vi "Camera Control.vi"(1 "i":i32) -> ()   [LabVIEW 2012]
uses:
  <vilib>/Rock Robotics/WPI/Joystick/WPI_JoystickGetSetRefNum.vi
  Robot Global Data.vi
panel:
  in  "Cam Y":dbl
  in  "Cam X":dbl
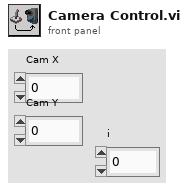
[diagram p1: front panel]
types:
  T1 = typedef "WPI_JoystickDevRef.ctl" = cluster{"Device":T2}
  T2 = typedef "WPI_JoystickDeviceEnum.ctl" = enum16{"USB 1", "USB 2", "USB 3", "USB 4", "Kinect 1", "Kinect 2"}
  T3 = typedef "WPI_JoystickButtonState.ctl" = cluster{"Button 1":bool, "Button 2":bool, "Button 3":bool, "Button 4":bool, "Button 5":bool, "Button 6":bool, "Button 7":bool, "Button 8":bool, "Button 9":bool, "Button 10":bool, "Button 11":bool, "Button 12":bool}
  T4 = cluster{"axis 1 (x)":dbl, "axis 2 (y)":dbl, "axis 3 (throttle)":dbl, "axis 4":dbl, "axis 5":dbl, "axis 6":dbl}
  T5 = typedef "WPI_ServoDeviceRef.ctl" = cluster{"DeviceStatus":errorcluster, "Digital Module":T6, "PWM Channel":T7, "DeadBand":T8}
  T6 = typedef "FPGA_TypedefDigitalModule.ctl" = enum16{"Digital Module 1", "Digital Module 2"}
  T7 = typedef "FPGA_DIOPWMChannel.ctl" = enum8{"PWM 1", "PWM 2", "PWM 3", "PWM 4", "PWM 5", "PWM 6", "PWM 7", "PWM 8", "PWM 9", "PWM 10", "Invalid"}
  T8 = typedef "WPI_PWMDeadband.ctl" = cluster{"Name":string, "maxPositivePwm":i32, "minPositivePwm":i32, "centerPwm":i32, "maxNegativePwm":i32, "minNegativePwm":i32, "angularRange":u16}
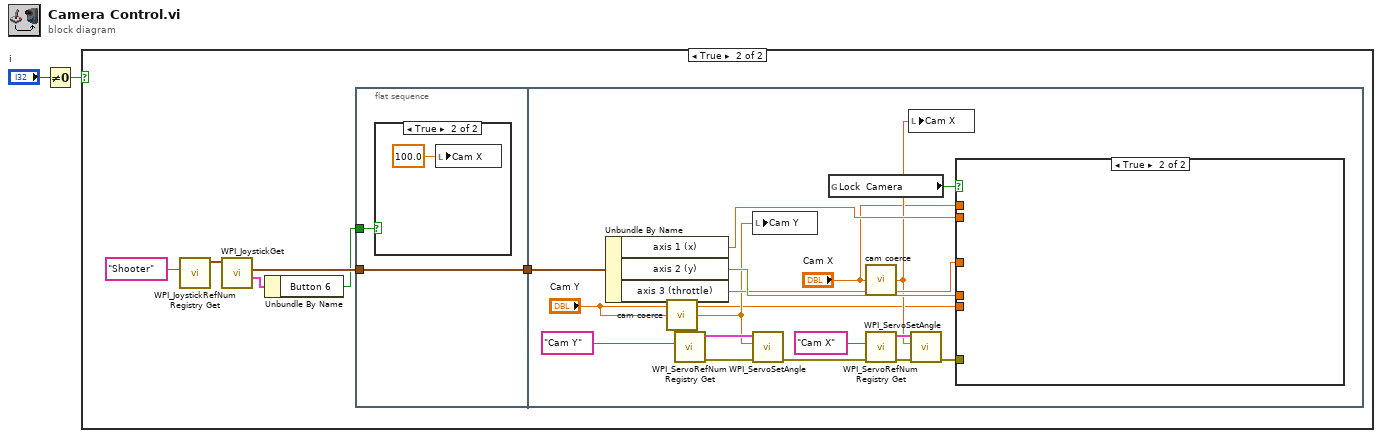
[diagram p0: block diagram]
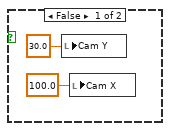
[diagram p2: hidden frame]
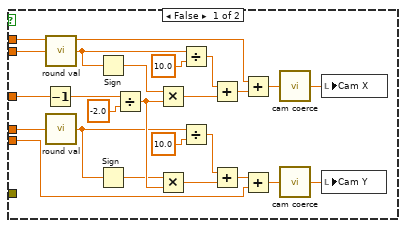
[diagram p4: hidden frame]
diagram:
  n1 = Not Equal To 0?(x="i") -> (x != 0?=w2:bool)
  n2 = case shown="True" w2 {
    frame False {
      n3 = local write "Cam Y"(30.0 ("Center y")) -> ()
      n4 = local write "Cam X"(100.0 ("Center x")) -> ()
    }
    frame True {
      n5 = call <vilib>:"WPI_JoystickRefNum Registry Get.vi"("refnum name"="Shooter") -> ("JoystickDevRef"=w9:T1)  [unwired: 1 in, 9 out]
      n6 = call <vilib>:"WPI_JoystickGet.vi"("JoystickDevRef"=w9) -> ("Buttons"=w7:T3, "Axes"=w8:T4)  [unwired: 1 in, 4 out]
      n7 = Unbundle By Name(w7) -> ("Button 6"=w5:bool)
      n8 = flat-sequence {
        tunnel: w8 -> [w12]
        tunnel: [w12] -> w6
        tunnel: w5 -> [w11]
        tunnel: w6 -> [w30]
        frame #0 {
          n9 = case shown="True" w11 {
            frame False {
            }
            frame True {
              n10 = local write "Cam X"(100.0 ("Cam X")) -> ()
            }
          }
        }
        frame #1 {
          n11 = Unbundle By Name(w30) -> ("axis 1 (x)"=w24:dbl, "axis 2 (y)"=w23:dbl, "axis 3 (throttle)"=w22:dbl)
          n12 = call "cam coerce.vi"("x"="Cam Y") -> ("coerced(x)"=w20:dbl)
          n13 = call <vilib>:"WPI_ServoRefNum Registry Get.vi"("refnum name"="Cam Y") -> ("error out"=w15:errorcluster, "ServoDeviceRef"=w27:T5)  [unwired: 9 in]
          n14 = local write "Cam Y"(w20) -> ()
          n15 = call <vilib>:"WPI_ServoSetAngle.vi"("error in (no error)"=w15, "Angle"=w20, "ServoDeviceRef"=w27) -> ("error out"=w14:errorcluster)  [unwired: 7 in, 1 out]
          n16 = global read "Robot Global Data.vi" "Lock  Camera"() -> (w29:bool)
          n17 = call "cam coerce.vi"("x"="Cam X") -> ("coerced(x)"=w21:dbl)
          n18 = call <vilib>:"WPI_ServoRefNum Registry Get.vi"("error in (no error)"=w14, "refnum name"="Cam X") -> ("error out"=w16:errorcluster, "ServoDeviceRef"=w25:T5)  [unwired: 8 in]
          n19 = local write "Cam X"(w21) -> ()
          n20 = call <vilib>:"WPI_ServoSetAngle.vi"("error in (no error)"=w16, "Angle"=w21, "ServoDeviceRef"=w25) -> ("error out"=w17:errorcluster)  [unwired: 7 in, 1 out]
          n21 = case shown="True" w29 {
            tunnel: w24 -> [w48 _]
            tunnel: w23 -> [w47 _]
            tunnel: w22 -> [w54 _]
            tunnel: "Cam Y" -> [w36 _]
            tunnel: "Cam X" -> [w35 _]
            tunnel: w17 -> [_ _]
            frame False {
              n22 = Decrement(x=w54) -> (x-1=w53:dbl)
              n23 = call "round val.vi"("num in"=w48) -> ("num out"=w46:dbl)
              n24 = call "round val.vi"("num in"=w47) -> ("num out"=w39:dbl)
              n25 = Sign(1:w46) -> (0:w50:dbl)
              n26 = Sign(1:w39) -> (0:w49:dbl)
              n27 = Divide(x=w53, y=-2.0) -> (x/y=w51:dbl)
              n28 = Multiply(x=w50, y=w51) -> (x*y=w43:dbl)
              n29 = Multiply(x=w49, y=w51) -> (x*y=w40:dbl)
              n30 = Divide(x=w46, y=10.0) -> (x/y=w44:dbl)
              n31 = Divide(x=w39, y=10.0) -> (x/y=w41:dbl)
              n32 = Add(x=w44, y=w43) -> (x+y=w38:dbl)
              n33 = Add(x=w41, y=w40) -> (x+y=w37:dbl)
              n34 = Add(x=w35, y=w38) -> (x+y=w32:dbl)
              n35 = Add(x=w37, y=w36) -> (x+y=w34:dbl)
              n36 = call "cam coerce.vi"("x"=w32) -> ("coerced(x)"=w31:dbl)
              n37 = call "cam coerce.vi"("x"=w34) -> ("coerced(x)"=w33:dbl)
              n38 = local write "Cam X"(w31) -> ()
              n39 = local write "Cam Y"(w33) -> ()
            }
            frame True {
            }
          }
        }
      }
    }
  }
